vi "Epoch Library -- VI Tree.vi"() -> ()   [LabVIEW 2017]
uses:
  Epochs -- enum.ctl
  formatter.iso8601/ISO8601 Date Formats.ctl
  Timestamp Compare Units -- enum.ctl
  formatter.iso8601/DateTime.ISO8601.lvclass
  C:/Users/patrick/Documents/GitHub/Epoch-Time/source/formatter/DateTimeFormatter.lvclass
  formatter.rfc5322/DateTime.RFC5322.lvclass
  epoch/Epoch.lvclass
  epoch.UTC/Epoch.UTC.lvclass
  epoch.GPS/Epoch.GPS.lvclass
  C:/Users/patrick/Documents/GitHub/Epoch-Time/source/epoch/Epoch.lvclass
  epoch.UNIX/Epoch.UNIX.lvclass
  formatter.iso8601/DateTime.ISO8601.lvclass/DateTime.ISO8601.ctl
  isLeapYear (timestamp).vi
  isLeapYear (integer).vi
  formatter/DateTimeFormatter.lvclass
panel:
  out "ISO String Comparison":bool
  out "is 10/14 in Daylight Savings?":bool
  out "Valid RFC5332 Internet Date":bool
  out "UNIX Conversion":bool
  out "UNIX Time (s)":i64
  out "GPS Time (s)":i64
  out "GPS Conversion":bool
  out "RFC5322 Email DateTime String":string
  out "Timestamp":timestamp
  out "ISO Strings":string[](array[string])
  out "timestamps":timestamp[](array[timestamp]) format="%<%.3X %x>T"
  out "Fractional Seconds":dbl[](array[numeric])
  out "Epoch Times (s)":i64[](array[numeric])
  out "Epochs":T1[](array[typedef])=[enum."Local", enum."UTC", enum."Unix", enum."GPS"]
  out "is 2021 a Leap Year?":bool
  out "ISO Week-Day Notation":bool
  out "ISO DateTime Notation":bool
  out "ISO8601 UTC DateTime String":string
  out "Valid RFC3339 Dates":bool
  out "Valid ISO Dates":bool
  out "is 2020 a Leap Year?":bool
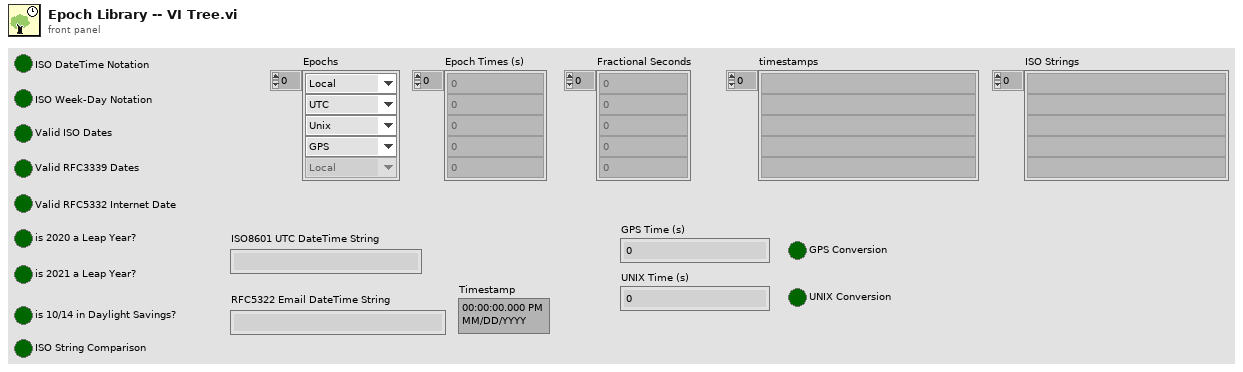
[diagram p1: front panel]
types:
  T1 = typedef "Epochs -- enum.ctl" = enum16{"Local", "UTC", "Unix", "GPS"}
  T2 = typedef "ISO8601 Date Formats.ctl" = enum16{"UTC Date-Time", "ISO Time", "Date", "Calendar Month", "Week", "Week-Day", "Month-Day", "Ordinal Date"}
  T3 = typedef "Timestamp Compare Units -- enum.ctl" = enum16{"week", "day", "hour", "minute", "second", "millisecond", "microsecond", "nanosecond"}
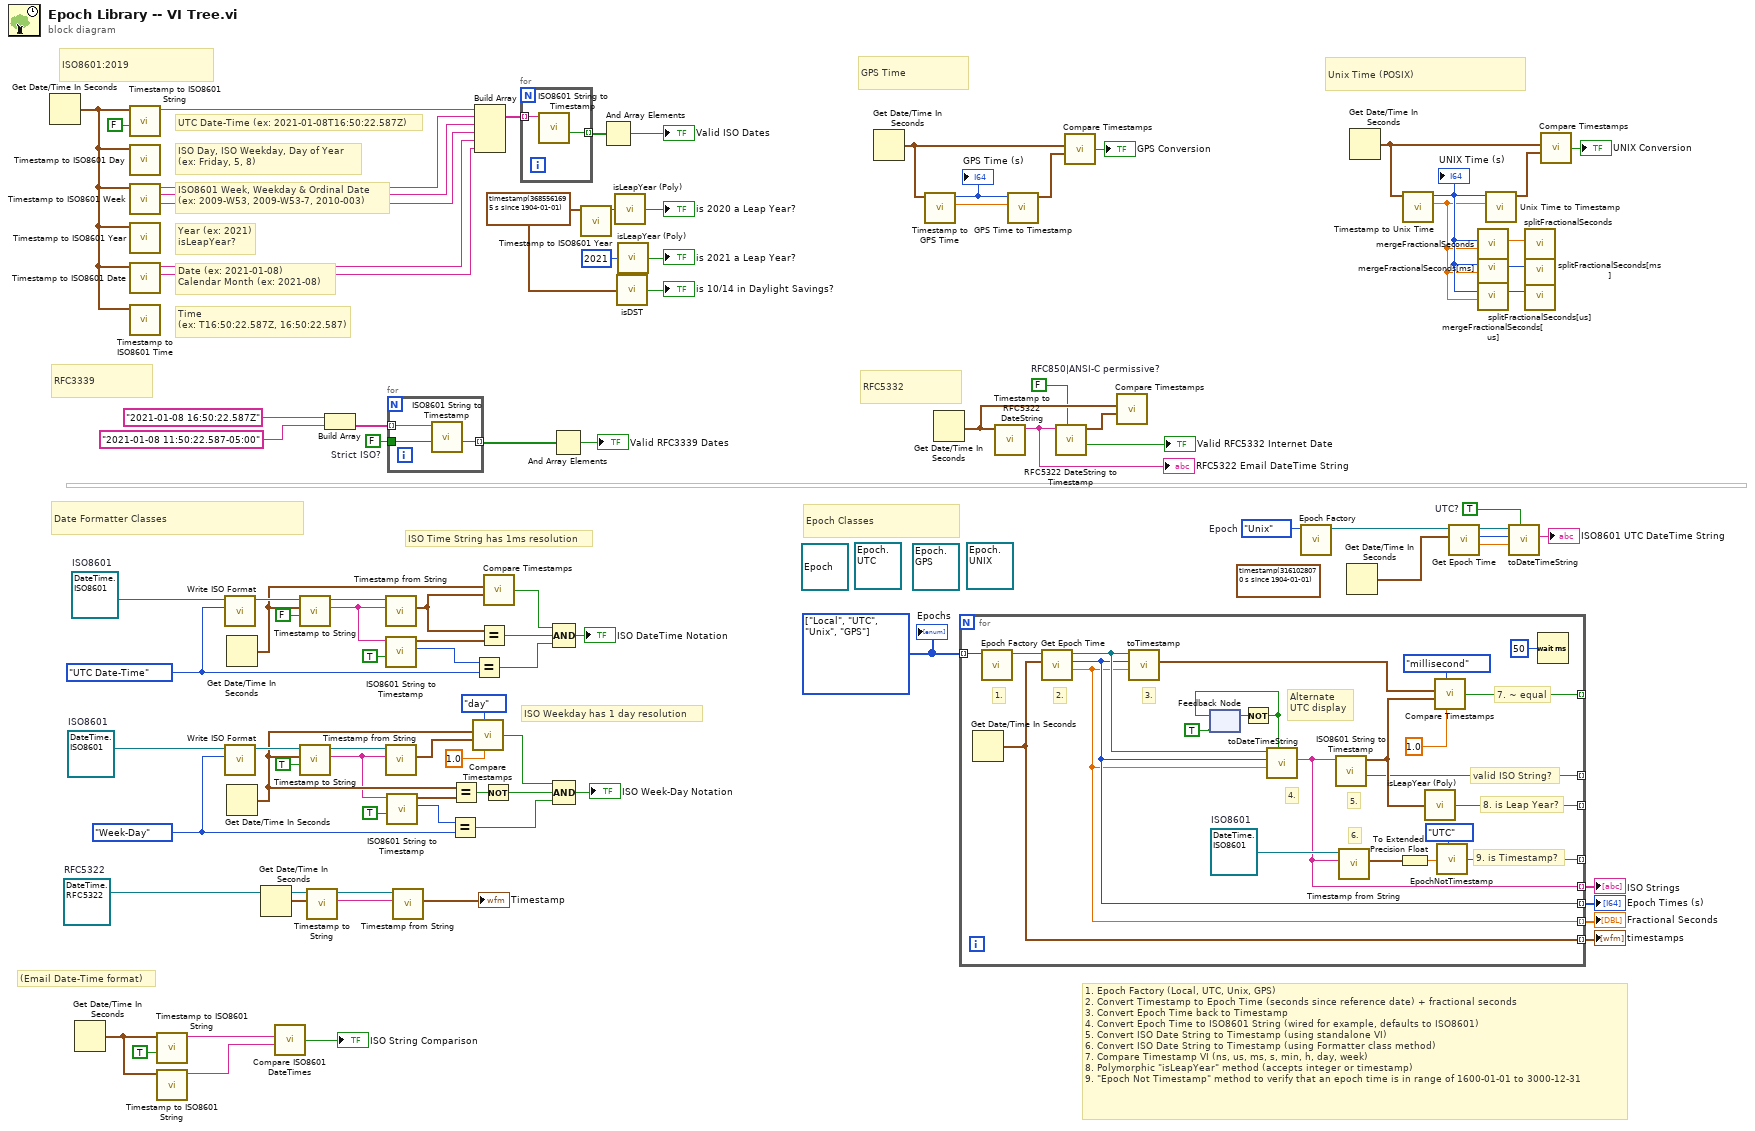
[diagram p0: block diagram]
diagram:
  w18 = FALSE  # RFC850|ANSI-C permissive?
  (unwired) refnum<class "Epoch.UNIX.lvclass"> refnum ("Epoch.UNIX.lvclass")
  (unwired) refnum<class "Epoch.GPS.lvclass"> refnum ("Epoch.GPS.lvclass")
  (unwired) refnum<class "Epoch.UTC.lvclass"> refnum ("Epoch.UTC.lvclass")
  (unwired) refnum<class "Epoch.lvclass"> refnum ("Epoch.lvclass")
  w30 = T1[] [enum."Local", enum."UTC", enum."Unix", enum."GPS"] items=["Local", "UTC", "Unix", "GPS"]
  w31 = TRUE  # UTC?
  (unwired) timestamp(3161028070.7687225 s since 1904-01-01) ("Timestamp (now)")
  w37 = Epochs_--_enum."Unix"  # Epoch
  w25 = timestamp(3685561695.389 s since 1904-01-01) ("Timestamp (now)")
  w61 = FALSE  # Strict ISO?
  w71 = refnum<class "DateTime.RFC5322.lvclass"> refnum  # RFC5322
  w87 = ISO8601_Date_Formats."Week-Day" ("ISO Format")
  w86 = refnum<class "DateTime.ISO8601.lvclass"> refnum  # ISO8601
  w94 = ISO8601_Date_Formats."UTC Date-Time" ("ISO Format")
  w95 = refnum<class "DateTime.ISO8601.lvclass"> refnum  # ISO8601
  # "Time\n(ex: T16:50:22.587Z, 16:50:22.587)"
  # "Epoch Classes"
  # "1. Epoch Factory (Local, UTC, Unix, GPS)\n2. Convert Timestamp to Epoch Time (seconds since reference date) + fractional seconds\n3. Convert Epoch Time back to Timestamp\n4. Convert Epoch Time to ISO8601 String (wired for example, defaults to ISO8601)\n5. Convert ISO Date String to Timestamp (using standalone VI)\n6. Convert ISO Date String to Timestamp (using Formatter class method)\n7. Compare Timestamp VI (ns, us, ms, s, min, h, day, week)\n8. Polymorphic \"isLeapYear\" method (accepts integer or timestamp)\n9. \"Epoch Not Timestamp\" method to verify that an epoch time is in range of 1600-01-01 to 3000-12-31"
  # "Date Formatter Classes"
  # "Unix Time (POSIX)"
  # "GPS Time"
  # "ISO8601:2019"
  # "Date (ex: 2021-01-08)\nCalendar Month (ex: 2021-08)"
  # "Year (ex: 2021)\nisLeapYear?"
  # "ISO8601 Week, Weekday & Ordinal Date\n(ex: 2009-W53, 2009-W53-7, 2010-003)"
  # "ISO Day, ISO Weekday, Day of Year\n(ex: Friday, 5, 8)"
  # "UTC Date-Time (ex: 2021-01-08T16:50:22.587Z)"
  # "RFC3339"
  # "RFC5332"
  # "(Email Date-Time format)"
  # "ISO Weekday has 1 day resolution"
  # "ISO Time String has 1ms resolution"
  n1 = Get Date/Time In Seconds() -> (seconds since 1Jan1904=w2:timestamp)
  n2 = Get Date/Time In Seconds() -> (seconds since 1Jan1904=w8:timestamp)
  n3 = call "Timestamp to ISO8601 String.vi"("UTC? (F)"=FALSE, "Timestamp (now)"=w2) -> ("ISO8601 String"=w15:string)  [unwired: 9 in]
  n4 = call "Timestamp to ISO8601 Day.vi"("Timestamp (now)"=w2) -> ()  [unwired: 8 in, 3 out]
  n5 = call "Timestamp to ISO8601 Week.vi"("Timestamp (now)"=w2) -> ("ISO8601 Ordinal Date"=w55:string, "ISO8601 Weekday"=w56:string, "ISO8601 Week"=w57:string)  [unwired: 8 in]
  n6 = call "Timestamp to ISO8601 Year.vi"("Timestamp (now)"=w2) -> ()  [unwired: 9 in, 2 out]
  n7 = call "Timestamp to ISO8601 Date.vi"("Timestamp (now)"=w2) -> ("ISO8601 Calendar Month"=w53:string, "ISO8601 Date"=w54:string)  [unwired: 9 in]
  n8 = call "Timestamp to ISO8601 Time.vi"("Timestamp (now)"=w2) -> ()  [unwired: 10 in, 1 out]
  n9 = call "Timestamp to ISO8601 String.vi"("UTC? (F)"=TRUE, "Timestamp (now)"=w8) -> ("ISO8601 String"=w9:string)  [unwired: 9 in]
  n10 = call "Timestamp to ISO8601 String.vi"("Timestamp (now)"=w8) -> ("ISO8601 String"=w7:string)  [unwired: 10 in]
  n11 = call "Write ISO Format.vi"("ISO Format"=w94, "DateTime.ISO8601 in"=w95) -> ("DateTime.ISO8601 out"=w96:refnum<class "DateTime.ISO8601.lvclass">)  [unwired: 9 in]
  n12 = call "Write ISO Format.vi"("ISO Format"=w87, "DateTime.ISO8601 in"=w86) -> ("DateTime.ISO8601 out"=w85:refnum<class "DateTime.ISO8601.lvclass">)  [unwired: 9 in]
  n13 = Get Date/Time In Seconds() -> (seconds since 1Jan1904=w73:timestamp)
  n14 = Get Date/Time In Seconds() -> (seconds since 1Jan1904=w83:timestamp)
  n15 = Get Date/Time In Seconds() -> (seconds since 1Jan1904=w69:timestamp)
  n16 = call "Compare ISO8601 DateTimes.vi"("ISO8601 DateTime (1)"=w9, "ISO8601 DateTime (2)"=w7) -> ("Equal?"=→"ISO String Comparison":bool)  [unwired: 6 in]
  n17 = call "Timestamp to String.vi"("UTC? (F)"=FALSE, "Timestamp (now)"=w73, "DateTimeFormatter in"=w96) -> ("DateTime String"=w6:string, "DateTimeFormatter out"=w97:refnum<class "DateTime.ISO8601.lvclass">)  [unwired: 6 in, 1 out]
  n18 = call "Timestamp to String.vi"("UTC? (F)"=TRUE, "Timestamp (now)"=w83, "DateTimeFormatter in"=w85) -> ("DateTime String"=w14:string, "DateTimeFormatter out"=w84:refnum<class "DateTime.ISO8601.lvclass">)  [unwired: 6 in, 1 out]
  n19 = call "Timestamp to String.vi"("Timestamp (now)"=w69, "DateTimeFormatter in"=w71) -> ("DateTime String"=w70:string, "DateTimeFormatter out"=w72:refnum<class "DateTime.RFC5322.lvclass">)  [unwired: 7 in, 1 out]
  n20 = Build Array("2021-01-08 16:50:22.587Z" ("x"), "2021-01-08 11:50:22.587-05:00" ("x")) -> (w64:string[])
  n21 = call "Timestamp from String.vi"("DateTime String"=w6, "DateTimeFormatter in"=w97) -> ("Timestamp"=w74:timestamp)  [unwired: 7 in, 2 out]
  n22 = call "ISO8601 String to Timestamp.vi"("Strict ISO? (T)"=TRUE, "ISO8601 String"=w6) -> ("ISO Format"=w4:T2, "Timestamp"=w3:timestamp)  [unwired: 7 in, 1 out]
  n23 = call "Timestamp from String.vi"("DateTime String"=w14, "DateTimeFormatter in"=w84) -> ("Timestamp"=w82:timestamp)  [unwired: 7 in, 2 out]
  n24 = call "ISO8601 String to Timestamp.vi"("Strict ISO? (T)"=TRUE, "ISO8601 String"=w14) -> ("ISO Format"=w12:T2, "Timestamp"=w11:timestamp)  [unwired: 7 in, 1 out]
  n25 = for {
    tunnel: w64 -> [w100] mode=indexing
    tunnel: [w98] -> w63 mode=indexing
    tunnel: w61 -> [w99]
    n26 = call "ISO8601 String to Timestamp.vi"("Strict ISO? (T)"=w99, "ISO8601 String"=w100) -> ("valid?"=w98:bool)  [unwired: 7 in, 2 out]
  }
  n27 = call "Timestamp from String.vi"("DateTime String"=w70, "DateTimeFormatter in"=w72) -> ("Timestamp"=→"Timestamp":timestamp)  [unwired: 7 in, 2 out]
  n28 = Equal?(x=w12, y=w87) -> (x = y?=w89:bool)
  n29 = Equal?(x=w83, y=w11) -> (x = y?=w88:bool)
  n30 = call "Compare Timestamps.vi"("Unit (ms)"=Timestamp_Compare_Units_--_enum."day" ("Unit (second)"), "timestamp (1)"=w83, "timestamp (2)"=w82, "Resolution (in selected unit)"=1.0) -> ("Equal?"=w81:bool)  [unwired: 4 in]
  n31 = Equal?(x=w4, y=w94) -> (x = y?=w92:bool)
  n32 = Build Array(w15, w57, w56, w55, w54, w53) -> (w52:string[])
  n33 = Equal?(x=w74, y=w3) -> (x = y?=w93:bool)
  n34 = Not(x=w88) -> (.not. x?=w80:bool)
  n35 = call "Compare Timestamps.vi"("timestamp (1)"=w73, "timestamp (2)"=w74) -> ("Equal?"=w75:bool)  [unwired: 6 in]
  n36 = for {
    tunnel: w52 -> [w102] mode=indexing
    tunnel: [w101] -> w51 mode=indexing
    n37 = call "ISO8601 String to Timestamp.vi"("ISO8601 String"=w102) -> ("valid?"=w101:bool)  [unwired: 8 in, 2 out]
  }
  n38 = And Array Elements(Boolean array=w63) -> (logical AND=→"Valid RFC3339 Dates":bool)
  n39 = Compound Arithmetic op=AND(w75, w93, w92) -> (→"ISO DateTime Notation":bool)
  n40 = Compound Arithmetic op=AND(w81, w80, w89) -> (→"ISO Week-Day Notation":bool)
  n41 = call "Timestamp to ISO8601 Year.vi"("Timestamp (now)"=w25) -> ("year"=w50:i32)  [unwired: 9 in, 1 out]
  n42 = And Array Elements(Boolean array=w51) -> (logical AND=→"Valid ISO Dates":bool)
  n43 = call-poly "isLeapYear (Poly).vi"("Year (0: this year)"=w50) -> ("is Leap Year?"=→"is 2020 a Leap Year?":bool)  [unwired: 8 in]
  n44 = call "isDST.vi"("timestamp (now)"=w25) -> ("is DST?"=→"is 10/14 in Daylight Savings?":bool)  [unwired: 8 in]
  n45 = call-poly "isLeapYear (Poly).vi"("Year (0: this year)"=2021) -> ("is Leap Year?"=→"is 2021 a Leap Year?":bool)  [unwired: 8 in]
  n46 = Get Date/Time In Seconds() -> (seconds since 1Jan1904=w44:timestamp)
  n47 = call "Timestamp to GPS Time.vi"("Timestamp (now)"=w44) -> ("Fractional Second"=w42:dbl, "GPS Time (s)"=w41:i64)  [unwired: 9 in]
  "GPS Time (s)" <- w41
  n48 = Get Date/Time In Seconds() -> (seconds since 1Jan1904=w65:timestamp)
  n49 = for {
    tunnel: w30 -> [w125] mode=indexing
    tunnel: [w121] -> _ mode=indexing
    tunnel: [w103] -> _ mode=indexing
    tunnel: [w118] -> _ mode=indexing
    tunnel: [w115] -> _ mode=indexing
    tunnel: [w114] -> w29 mode=indexing
    tunnel: [w113] -> w28 mode=indexing
    tunnel: [w108] -> w27 mode=indexing
    tunnel: [w105] -> w26 mode=indexing
    w119 = refnum<class "DateTime.ISO8601.lvclass"> refnum  # ISO8601
    # "Alternate\nUTC display"
    # "6."
    # "5."
    # "9. is Timestamp?"
    # "8. is Leap Year?"
    # "valid ISO String?"
    # "7. ~ equal"
    # "4."
    # "3."
    # "2."
    # "1."
    n50 = Get Date/Time In Seconds() -> (seconds since 1Jan1904=w108:timestamp)
    n51 = call "Epoch Factory.vi"("Epoch (Local System)"=w125) -> ("Epoch object"=w124:refnum<class "Epoch.lvclass">)  [unwired: 10 in]
    n52 = call "Get Epoch Time.vi"("Timestamp (now)"=w108, "Epoch (Local)"=w124) -> ("Fractional Second"=w113:dbl, "Epoch Time (s)"=w114:i64, "Epoch out"=w120:refnum<class "Epoch.lvclass">)  [unwired: 7 in]
    n53 = call-dynamic "toTimestamp.vi"("Fractional Second"=w113, "Epoch Time (s)"=w114, "Epoch (Local)"=w120) -> ("Timestamp"=w107:timestamp)  [unwired: 6 in, 2 out]
    n54 = feedback #1(TRUE) -> (w110:bool)
    n55 = Not(x=w110) -> (.not. x?=w109:bool)
    n56 = feedback-in #1(w109) -> ()
    n57 = call "toDateTimeString.vi"("UTC? (F)"=w109, "Fractional Second"=w113, "Epoch Time (s)"=w114, "Epoch"=w120) -> ("DateTime string"=w105:string)  [unwired: 5 in, 2 out]
    n58 = call "ISO8601 String to Timestamp.vi"("ISO8601 String"=w105) -> ("valid?"=w103:bool, "Timestamp"=w104:timestamp)  [unwired: 8 in, 1 out]
    n59 = call "Timestamp from String.vi"("DateTime String"=w105, "DateTimeFormatter in"=w119) -> ("Timestamp"=w106:timestamp)  [unwired: 7 in, 2 out]
    n60 = To Extended Precision Float(1:w106) -> (0:w117:ext)
    n61 = call-poly "isLeapYear (Poly).vi"("timestamp (now)"=w104) -> ("is Leap Year?"=w118:bool)  [unwired: 8 in]
    n62 = call "Compare Timestamps.vi"("Unit (ms)"=Timestamp_Compare_Units_--_enum."millisecond" ("Unit (second)"), "timestamp (1)"=w107, "timestamp (2)"=w104, "Resolution (in selected unit)"=1.0) -> ("Equal?"=w121:bool)  [unwired: 4 in]
    n63 = call "EpochNotTimestamp.vi"("Epoch (UTC)"=Epochs_--_enum."UTC", "Epoch Time"=w117) -> ("Not a Timestamp?"=w115:bool)  [unwired: 7 in]
    n64 = Wait (ms)(milliseconds to wait=u32 50) -> ()  [unwired: 1 out]
  }
  "Epoch Times (s)" <- w29
  "Fractional Seconds" <- w28
  "timestamps" <- w27
  "ISO Strings" <- w26
  n65 = call "Timestamp to RFC5322 DateString.vi"("Timestamp (now)"=w65) -> ("RFC5322 Date String"=w67:string)  [unwired: 10 in]
  "RFC5322 Email DateTime String" <- w67
  n66 = call "GPS Time to Timestamp.vi"("Fractional Second"=w42, "GPS Time (s)"=w41) -> ("Timestamp"=w43:timestamp)  [unwired: 8 in, 1 out]
  n67 = call "RFC5322 DateString to Timestamp.vi"("RFC850|ANSI-C permissive?"=w18, "RFC5322 String"=w67) -> ("valid?"=→"Valid RFC5332 Internet Date":bool, "Timestamp"=w66:timestamp)  [unwired: 7 in, 1 out]
  n68 = call "Compare Timestamps.vi"("timestamp (1)"=w44, "timestamp (2)"=w43) -> ("Equal?"=→"GPS Conversion":bool)  [unwired: 6 in]
  n69 = call "Compare Timestamps.vi"("timestamp (1)"=w65, "timestamp (2)"=w66) -> ()  [unwired: 6 in, 1 out]
  n70 = call "Epoch Factory.vi"("Epoch (Local System)"=w37) -> ("Epoch object"=w36:refnum<class "Epoch.lvclass">)  [unwired: 10 in]
  n71 = Get Date/Time In Seconds() -> (seconds since 1Jan1904=w1:timestamp)
  n72 = Get Date/Time In Seconds() -> (seconds since 1Jan1904=w39:timestamp)
  n73 = call "Timestamp to Unix Time.vi"("Timestamp (now)"=w39) -> ("Fractional Second"=w21:dbl, "Unix Time (s)"=w22:i64)  [unwired: 9 in]
  "UNIX Time (s)" <- w22
  n74 = call "Get Epoch Time.vi"("Timestamp (now)"=w1, "Epoch (Local)"=w36) -> ("Fractional Second"=w35:dbl, "Epoch Time (s)"=w34:i64, "Epoch out"=w33:refnum<class "Epoch.lvclass">)  [unwired: 7 in]
  n75 = call "mergeFractionalSeconds.vi"("Fractional Second"=w21, "(Integer) Time (s)"=w22) -> ("(Float) Time (s)"=w23:dbl)  [unwired: 8 in, 1 out]
  n76 = call "mergeFractionalSeconds[ms].vi"("Fractional Second"=w21, "(Integer) Time (s)"=w22) -> ("(Integer) Time (ms)"=w19:i64)  [unwired: 8 in, 1 out]
  n77 = call "mergeFractionalSeconds[us].vi"("Fractional Second"=w21, "(Integer) Time (s)"=w22) -> ("(Integer) Time (us)"=w20:i64)  [unwired: 8 in, 1 out]
  n78 = call "Unix Time to Timestamp.vi"("Fractional Second"=w21, "Unix Time (s)"=w22) -> ("Timestamp"=w38:timestamp)  [unwired: 8 in, 1 out]
  n79 = call "toDateTimeString.vi"("UTC? (F)"=w31, "Fractional Second"=w35, "Epoch Time (s)"=w34, "Epoch"=w33) -> ("DateTime string"=→"ISO8601 UTC DateTime String":string)  [unwired: 5 in, 2 out]
  n80 = call "splitFractionalSeconds.vi"("(Float) Time (s)"=w23) -> ()  [unwired: 8 in, 3 out]
  n81 = call "splitFractionalSeconds[ms].vi"("(Integer) Time (ms)"=w19) -> ()  [unwired: 8 in, 3 out]
  n82 = call "splitFractionalSeconds[us].vi"("(Integer) Time (us)"=w20) -> ()  [unwired: 8 in, 3 out]
  n83 = call "Compare Timestamps.vi"("timestamp (1)"=w39, "timestamp (2)"=w38) -> ("Equal?"=→"UNIX Conversion":bool)  [unwired: 6 in]
  "Epochs" <- w30
